vi "GetGrphScaleNmGen.vi"(8 "ErrorIn(No Error)":errorcluster caption="entrée d'erreur (pas d'erreur)", 11 "GraphRef":refnum<vi>) -> (0 "sortie d'erreur":errorcluster, 2 "YScales":string[](array[string]), 3 "XScales":string[](array[string]), 4 "YScInd":i32[](array[numeric]), 5 "XScInd":i32[](array[numeric]))   [LabVIEW 2010]
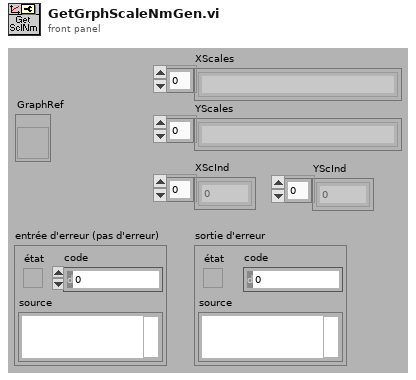
[diagram p1: front panel]
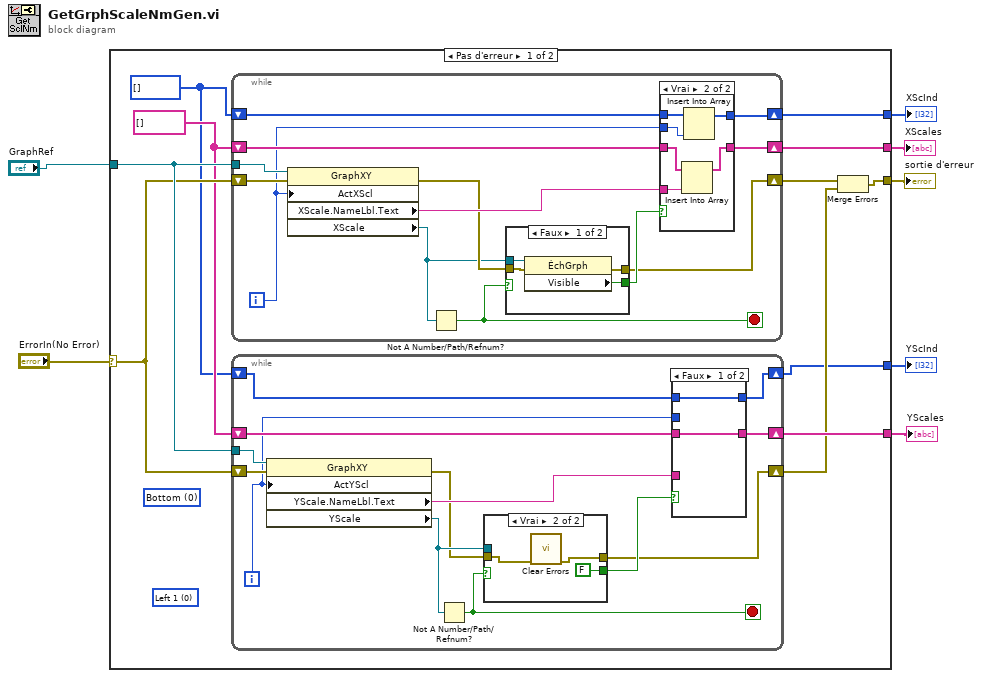
[diagram p0: block diagram]
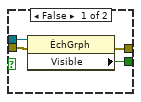
[diagram p2: hidden frame]
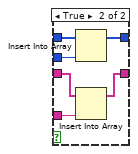
[diagram p3: hidden frame]
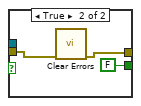
[diagram p4: hidden frame]
diagram:
  n1 = case shown="Pas d'erreur" "ErrorIn(No Error)" {
    selector: "ErrorIn(No Error)" -> [w16 w75]
    tunnel: [w13 w75] -> w6
    tunnel: [w18 _] -> w5
    tunnel: "GraphRef" -> [w17 _]
    tunnel: [w15 _] -> w3
    tunnel: [w9 _] -> w2
    tunnel: [w8 _] -> w1
    frame No Error {
      w10 = i32[] []
      (unwired) u16 0 items=["Bottom", "Top"]
      (unwired) u16 0 items=["Left 1", "Left 2", "Left 3", "Right 1", "Right 2", "Right 3"]
      w14 = string[] []
      n2 = while {
        tunnel: w17 -> [w59]
        shift-right: [w50] -> w12
        shift-left: w16 -> [w58]
        shift-right: [w56] -> w18
        shift-left: w14 -> [w55]
        shift-right: [w48] -> w9
        shift-left: w10 -> [w47]
        i -> [w49]
        stop <- w54 stop-if-true
        n3 = property class="GraphXY"(reference=w59, error in=w58, "ActXScl"=w49) -> (error out=w53:errorcluster, "XScale.NameLbl.Text"=w57:string, "XScale"=w52:refnum<vi>)  [unwired: 1 out]
        n4 = Not A Number/Path/Refnum?(number/path/refnum=w52) -> (NaN/Path/Refnum?=w54:bool)
        n5 = case shown="Faux" w54 {
          tunnel: w52 -> [w63 _]
          tunnel: w53 -> [w62 w65]
          tunnel: [w61 FALSE ("Visible")] -> w51
          tunnel: [w60 w64] -> w50
          frame False {
            n6 = property class="ÉchGrph"(reference=w63, error in=w62) -> (error out=w60:errorcluster, "Visible"=w61:bool)  [unwired: 1 out]
          }
          frame True {
            n7 = call <vilib>:"Clear Errors.vi"("error in (no error)"=w65) -> ("error out"=w64:errorcluster)  [unwired: 6 in]
          }
        }
        n8 = case shown="Vrai" w51 {
          tunnel: w57 -> [_ w74]
          tunnel: [w68 w73] -> w56
          tunnel: w55 -> [w68 w72]
          tunnel: w49 -> [_ w69]
          tunnel: [w67 w71] -> w48
          tunnel: w47 -> [w67 w70]
          frame False {
          }
          frame True {
            n9 = Insert Into Array(array=w72, new element=w74) -> (w73:string[])  [unwired: 1 in]
            n10 = Insert Into Array(array=w70, new element=w69) -> (w71:i32[])  [unwired: 1 in]
          }
        }
      }
      n11 = while {
        tunnel: w17 -> [w31]
        shift-right: [w22] -> w11
        shift-left: w16 -> [w26]
        shift-right: [w29] -> w15
        shift-left: w14 -> [w28]
        shift-right: [w19] -> w8
        shift-left: w10 -> [w20]
        i -> [w21]
        stop <- w25 stop-if-true
        n12 = property class="GraphXY"(reference=w31, error in=w26, "ActYScl"=w21) -> (error out=w24:errorcluster, "YScale.NameLbl.Text"=w30:string, "YScale"=w27:refnum<vi>)  [unwired: 1 out]
        n13 = Not A Number/Path/Refnum?(number/path/refnum=w27) -> (NaN/Path/Refnum?=w25:bool)
        n14 = case shown="Vrai" w25 {
          tunnel: w27 -> [w35 _]
          tunnel: w24 -> [w34 w37]
          tunnel: [w33 FALSE ("Visible")] -> w23
          tunnel: [w32 w36] -> w22
          frame False {
            n15 = property class="ÉchGrph"(reference=w35, error in=w34) -> (error out=w32:errorcluster, "Visible"=w33:bool)  [unwired: 1 out]
          }
          frame True {
            n16 = call <vilib>:"Clear Errors.vi"("error in (no error)"=w37) -> ("error out"=w36:errorcluster)  [unwired: 6 in]
          }
        }
        n17 = case shown="Faux" w23 {
          tunnel: w30 -> [_ w46]
          tunnel: [w40 w45] -> w29
          tunnel: w28 -> [w40 w44]
          tunnel: w21 -> [_ w43]
          tunnel: w20 -> [w39 w42]
          tunnel: [w39 w41] -> w19
          frame False {
          }
          frame True {
            n18 = Insert Into Array(array=w42, new element=w43) -> (w41:i32[])  [unwired: 1 in]
            n19 = Insert Into Array(array=w44, new element=w46) -> (w45:string[])  [unwired: 1 in]
          }
        }
      }
      n20 = Merge Errors(w12, w11) -> (w13:errorcluster)
    }
    frame Error {
    }
  }
  "sortie d'erreur" <- w6
  "XScales" <- w5
  "YScales" <- w3
  "XScInd" <- w2
  "YScInd" <- w1
